vi "calc mods from center.vi"(8 "error in (no error)":errorcluster, 11 "pivot center":T1 {"Y" format="%.4g"; "X" format="%.4g"}) -> (0 "error out":errorcluster)   [LabVIEW 2023]
uses:
  ctrl defs/ctrl XY coord.ctl
  ctrl defs/ctrl swerve module.ctl
  Global odometry.vi
panel:
  out "PARK ANGLEs (deg)":dbl[](array[numeric])
  out "PARKING angle (deg)":dbl
  out "output to swerve module data":T2[](array[typedef]) {"corner wt (lbm)" format="%#.3f"; "POS" format="%.3g"; "coord wrt geom CTR"."Y" format="%.4g"; "coord wrt geom CTR"."X" format="%.4g"; "from pivot to module"."theta park (deg)" format="%.4g"; "from pivot to module"."theta spin (deg)" format="%.4g"; "from pivot to module"."theta (deg)" format="%.4g"; "from pivot to module"."R" format="%.4g"; "ABS" format="%.3g"; "target" format="%.3g"; "V" format="%.3g"}
  out "gem ctr to module":cluster{"geomX":dbl, "geomY":dbl}[](array[cluster])
  out "pivot to module":T1[](array[typedef]) {"Y" format="%.4g"; "X" format="%.4g"}
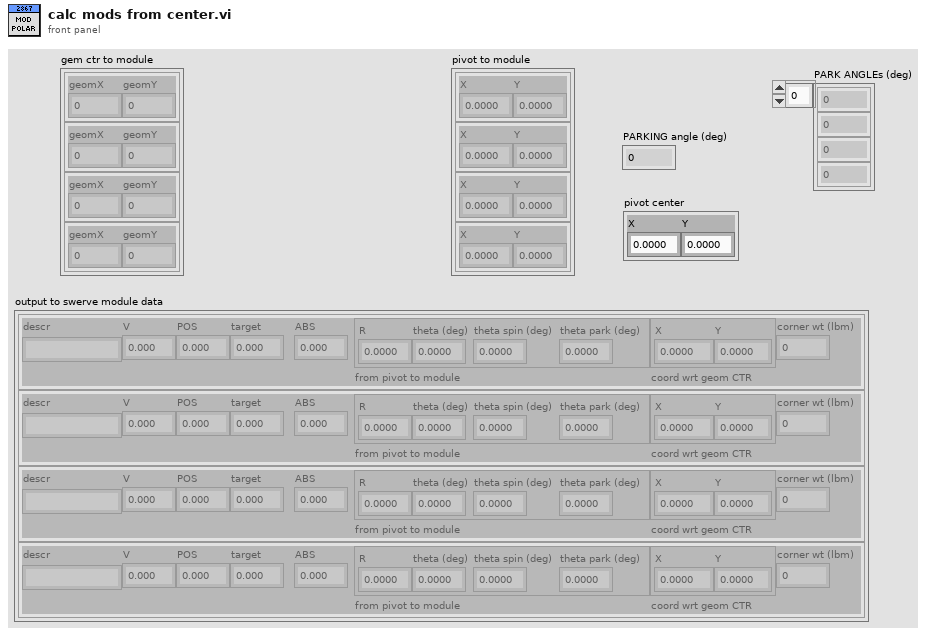
[diagram p1: front panel]
types:
  T1 = typedef "ctrl XY coord.ctl" = cluster{"X":dbl, "Y":dbl}
  T2 = typedef "ctrl swerve module.ctl" = cluster{"descr":string, "V":dbl, "POS":dbl, "target":dbl, "ABS":dbl, "from pivot to module":cluster{"R":dbl, "theta (deg)":dbl, "theta spin (deg)":dbl, "theta park (deg)":dbl}, "coord wrt geom CTR":cluster{"X":dbl, "Y":dbl}, "corner wt (lbm)":dbl}
  T3 = typedef "ctrl PARKING constants.ctl" = cluster{"angle (deg)":dbl, "%VBus":dbl}
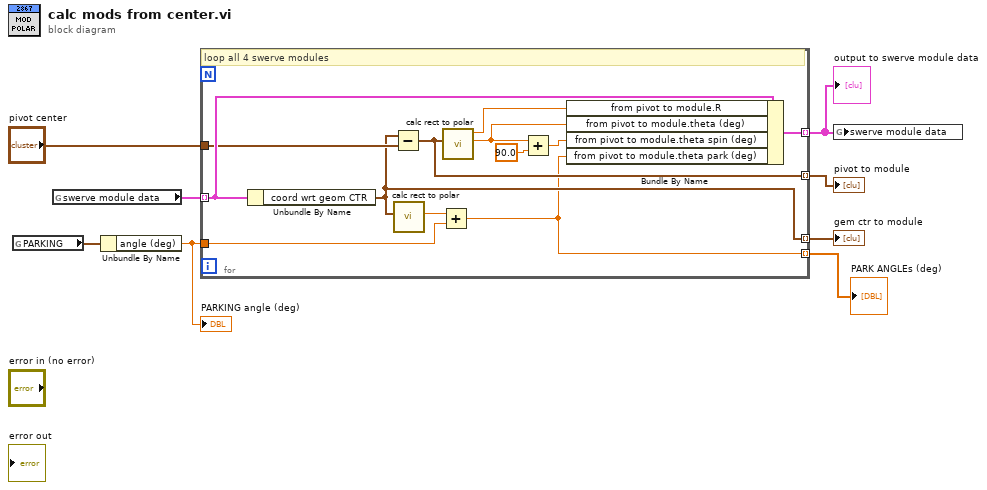
[diagram p0: block diagram]
diagram:
  n1 = global read "Global odometry.vi" "PARKING"() -> (w3:T3)
  n2 = global read "Global odometry.vi" "swerve module data"() -> (w8:T2[])
  n3 = Unbundle By Name(w3) -> ("angle (deg)"=w2:dbl)
  "PARKING angle (deg)" <- w2
  n4 = for {
    tunnel: w8 -> [w19] mode=indexing
    tunnel: [w20] -> w7 mode=indexing
    tunnel: "pivot center" -> [w16]
    tunnel: [w17] -> w6 mode=indexing
    tunnel: [w12] -> w5 mode=indexing
    tunnel: w2 -> [w10]
    tunnel: [w9] -> w1 mode=indexing
    # "loop all 4 swerve modules"
    n5 = Unbundle By Name(w19) -> ("coord wrt geom CTR"=w12:cluster{"X":dbl, "Y":dbl})
    n6 = Subtract(x=w12, y=w16) -> (x-y=w17:T1)
    n7 = call "calc rect to polar.vi"("XY"=w12) -> ("angle (deg)"=w11:dbl)  [unwired: 8 in, 2 out]
    n8 = Add(x=w11, y=w10) -> (x+y=w9:dbl)
    n9 = call "calc rect to polar.vi"("XY"=w17) -> ("angle (deg)"=w15:dbl, "Magnitude"=w18:dbl)  [unwired: 8 in, 1 out]
    n10 = Add(x=w15, y=90.0) -> (x+y=w14:dbl)
    n11 = Bundle By Name(cluster=w19, "from pivot to module.R"=w18, "from pivot to module.theta (deg)"=w15, "from pivot to module.theta spin (deg)"=w14, "from pivot to module.theta park (deg)"=w9) -> (w20:T2)
  }
  "pivot to module" <- w6
  "gem ctr to module" <- w5
  "output to swerve module data" <- w7
  "PARK ANGLEs (deg)" <- w1
  n12 = global write "Global odometry.vi" "swerve module data"(w7) -> ()
